vi "ViewInsertVI.vi"(9 "UpdateInsertableVI":T1[](array[typedef]), 10 "Name":string, 11 "TabControl in":refnum<vi>) -> ()   [LabVIEW 2020, in "MDI ViewManager.lvlib"]
uses:
  MDI ViewManager.lvlib
  Typedef/UpdateInsertableVICtl.ctl
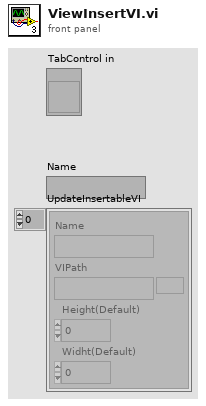
[diagram p1: front panel]
types:
  T1 = typedef "MDI ViewManager.lvlib/UpdateInsertableVICtl.ctl" = cluster{"Name":string, "VIPath":path, "Height(Default)":dbl, "Widht(Default)":dbl}
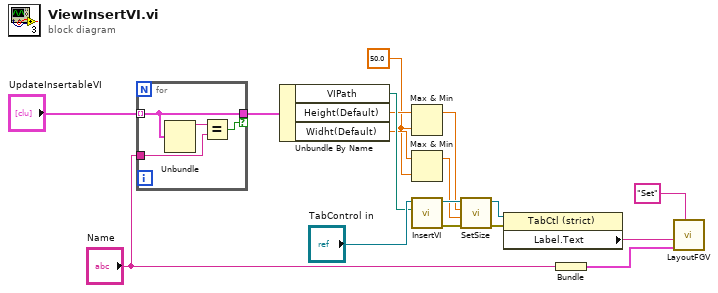
[diagram p0: block diagram]
diagram:
  w2 = 50.0 ("y")
  n1 = for {
    tunnel: "UpdateInsertableVI" -> [w18] mode=indexing
    tunnel: "Name" -> [w21]
    tunnel: [w18] -> w7 if=w19
    n2 = Unbundle(w18) -> ("Name"=w20:string)  [unwired: 3 out]
    n3 = Equal?(x=w20, y=w21) -> (x = y?=w19:bool)
  }
  n4 = Unbundle By Name(w7) -> ("VIPath"=w6:path, "Height(Default)"=w5:dbl, "Widht(Default)"=w3:dbl)
  n5 = Max & Min(x=w5, y=w2) -> (max(x,y)=w4:dbl)  [unwired: 1 out]
  n6 = Max & Min(x=w3, y=w2) -> (max(x,y)=w1:dbl)  [unwired: 1 out]
  n7 = call "InsertVI.vi"("VIPath"=w6, "TabControl in"="TabControl in") -> ("error out"=w9:errorcluster, "TabControl out"=w11:refnum<vi>)  [unwired: 8 in]
  n8 = call "SetSize.vi"("error in (no error)"=w9, "Widht"=w1, "Height"=w4, "TabControl in"=w11) -> ("error out"=w8:errorcluster, "reference out"=w10:refnum<vi>)  [unwired: 6 in]
  n9 = property class="TabCtl (strict)"(reference=w10, error in=w8) -> ("Label.Text"=w15:string)  [unwired: 2 out]
  n10 = Bundle("Name"="Name") -> (w14:cluster{"Name":string})  [unwired: 1 in]
  n11 = call "LayoutFGV.vi"("String"="Set", "Variant"=w14, "name"=w15) -> ()  [unwired: 9 in]
